vi "data insert.vi"(8 "error in (no error)":errorcluster, 9 "集成干预":bool, 10 "data":T1={"时间"=timestamp(0 s since 1904-01-01), "测量模式"="水样测试", "数据类型"="N", "检测值"=0.0, "单位"="mg/L", "数据标识"="N", "信号值"=0.0, "标样参考值"=0.0, "因子编码"="", "探头温度"=0.0, "LastTime"=timestamp(0 s since 1904-01-01)}, 11 "table in":string(combo)) -> (0 "error out":errorcluster)   [LabVIEW 2022 SP3, in "斯坦道多参数.lvlib"]
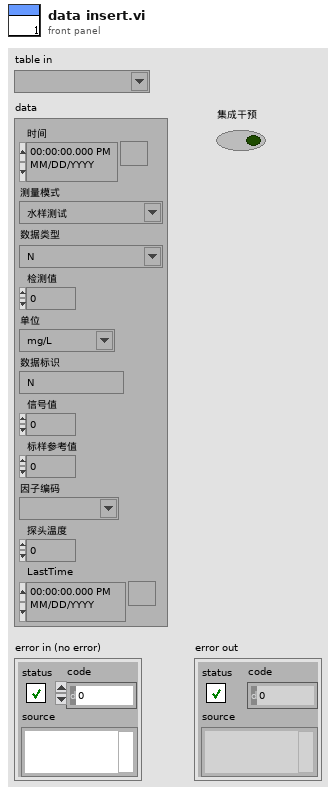
[diagram p1: front panel]
types:
  T1 = typedef "集成多参数单参数字段定义.ctl" = cluster{"时间":timestamp, "测量模式":string, "数据类型":string, "检测值":sgl, "单位":string, "数据标识":string, "信号值":sgl, "标样参考值":sgl, "因子编码":string, "探头温度":sgl, "LastTime":timestamp}
  T2 = typedef "集成干预字段定义.ctl" = cluster{"时间":timestamp, "参数":string, "数据类型":string, "集成干预测试浓度值":dbl, "集成干预前测试时间":timestamp, "集成干预前测试浓度值":dbl}
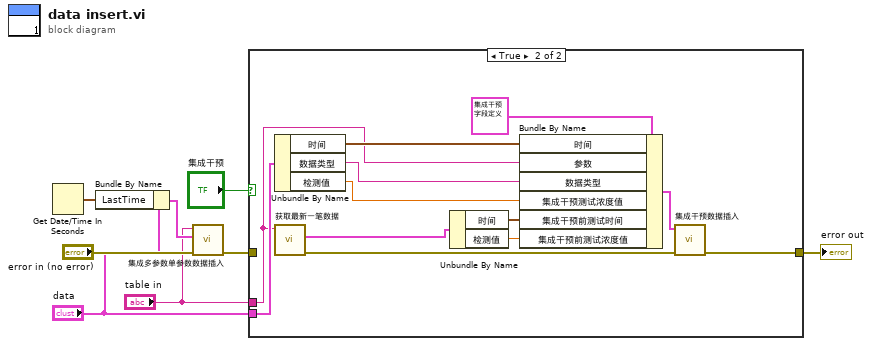
[diagram p0: block diagram]
diagram:
  n1 = Get Date/Time In Seconds() -> (seconds since 1Jan1904=w6:timestamp)
  n2 = Bundle By Name(cluster="data", "LastTime"=w6) -> (w7:T1)
  n3 = call "集成多参数单参数数据插入.vi"("Tabe Name"="table in", "data"=w7, "错误输入（无错误）"="error in (no error)") -> ("错误输出"=w4:errorcluster)  [unwired: 7 in]
  n4 = case shown="True" "集成干预" {
    tunnel: w4 -> [w9 _]
    tunnel: "table in" -> [_ w12]
    tunnel: [w9 w18] -> w2
    tunnel: "data" -> [_ w16]
    frame False {
    }
    frame True {
      n5 = Unbundle By Name(w16) -> ("时间"=w13:timestamp, "数据类型"=w11:string, "检测值"=w10:sgl)
      n6 = call "获取最新一笔数据.vi"("table"=w12) -> ("错误输出"=w17:errorcluster, "检测值"=w21:cluster{"时间":timestamp, "检测值":dbl})  [unwired: 8 in, 1 out]
      n7 = Unbundle By Name(w21) -> ("时间"=w15:timestamp, "检测值"=w14:dbl)
      n8 = Bundle By Name(cluster=T2 {"时间"=timestamp(0 s since 1904-01-01), "参数"="", "数据类型"="N", "集成干预测试浓度值"=0.0, "集成干预前测试时间"=timestamp(0 s since 1904-01-01), "集成干预前测试浓度值"=0.0} ("集成干预测试数据"), "时间"=w13, "参数"=w12, "数据类型"=w11, "集成干预测试浓度值"=w10, "集成干预前测试时间"=w15, "集成干预前测试浓度值"=w14) -> (w19:T2)
      n9 = call "集成干预数据插入.vi"("error in (no error)"=w17, "集成干预测试数据"=w19) -> ("error out"=w18:errorcluster)  [unwired: 9 in]
    }
  }
  "error out" <- w2
